vi "Initialize.vi"(0 "Gate Filter":bool, 1 "Gate Speed":dbl format="%.2f", 2 "Gate Dely":dbl format="%.2f", 3 "Gate Compliance (A)":dbl=0.001 format="%.2e", 4 "Drain Filter":bool, 5 "Drain Speed":dbl format="%.2f", 6 "Drain Delay":dbl format="%.2f", 7 "Drain Compliance (A)":dbl=0.001 format="%.2e") -> ()   [LabVIEW 2020]
panel:
  # "Initialize VI"
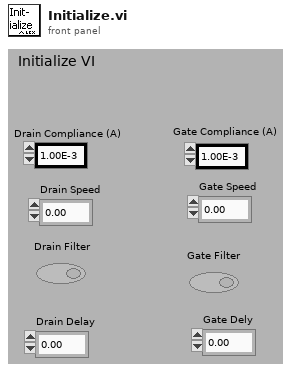
[diagram p1: front panel]
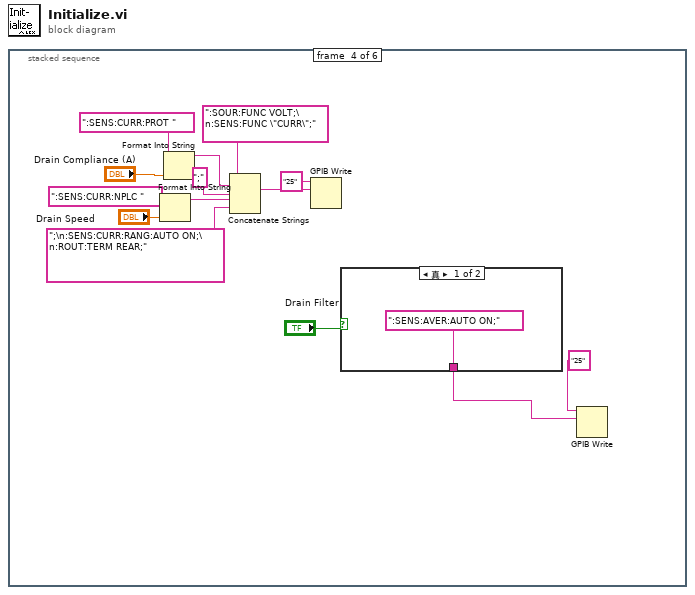
[diagram p0: block diagram]
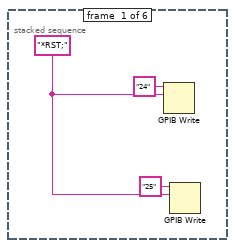
[diagram p2: hidden frame]
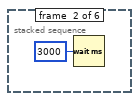
[diagram p3: hidden frame]
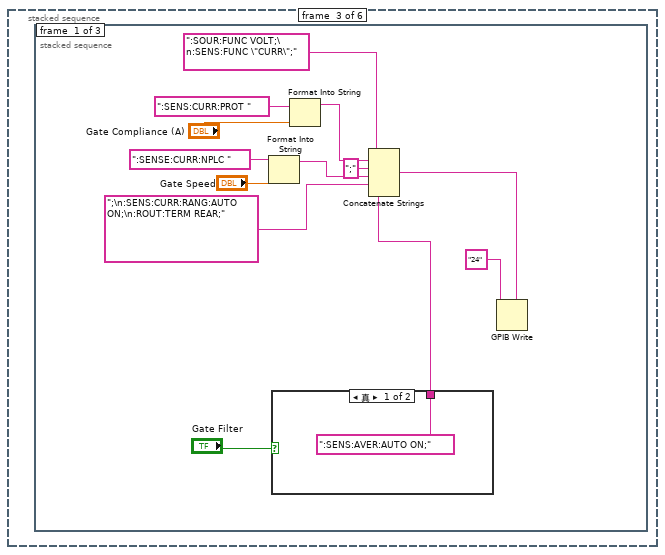
[diagram p4: hidden frame]
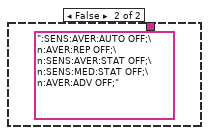
[diagram p5: hidden frame]
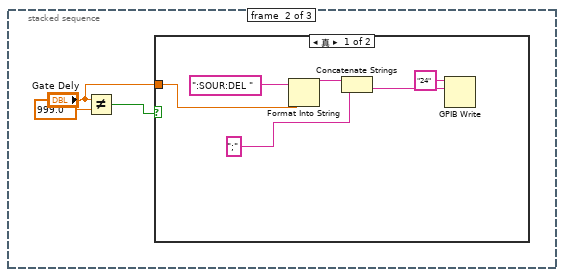
[diagram p6: hidden frame]
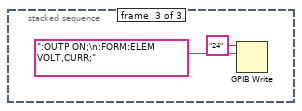
[diagram p8: hidden frame]
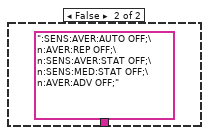
[diagram p9: hidden frame]
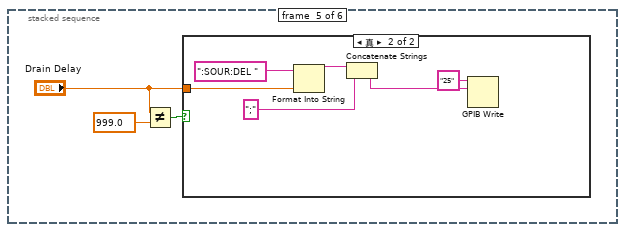
[diagram p10: hidden frame]
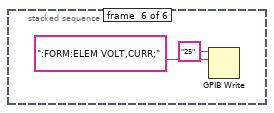
[diagram p12: hidden frame]
diagram:
  n1 = stacked-sequence {
    frame #0 {
      w1 = "*RST;"
      n2 = GPIB Write(0:"24" ("address string"), 1:w1) -> ()  [unwired: 3 in, 2 out]
      n3 = GPIB Write(0:"25" ("address string"), 1:w1) -> ()  [unwired: 3 in, 2 out]
    }
    frame #1 {
      n4 = Wait (ms)(milliseconds to wait=u32 3000) -> ()  [unwired: 1 out]
    }
    frame #2 {
      n5 = stacked-sequence {
        frame #0 {
          n6 = Format Into String(initial string=":SENSE:CURR:NPLC ", "Gate Speed") -> (resulting string=w6:string)  [unwired: 2 in, 1 out]
          n7 = case shown="真" "Gate Filter" {
            tunnel: [":SENS:AVER:AUTO ON;" ":SENS:AVER:AUTO OFF;\n:AVER:REP OFF;\n:SENS:AVER:STAT OFF;\n:SENS:MED:STAT OFF;\n:AVER:ADV OFF;"] -> w8
            frame True {
            }
            frame False {
            }
          }
          n8 = Format Into String(initial string=":SENS:CURR:PROT ", "Gate Compliance (A)") -> (resulting string=w13:string)  [unwired: 2 in, 1 out]
          n9 = Concatenate Strings(":SOUR:FUNC VOLT;\n:SENS:FUNC \"CURR\";", w13, ";" ("Substring"), w6, ";\n:SENS:CURR:RANG:AUTO ON;\n:ROUT:TERM REAR;", w8) -> (w15:string)
          n10 = GPIB Write(0:"24", 1:w15) -> ()  [unwired: 3 in, 2 out]
        }
        frame #1 {
          n11 = Not Equal?(x="Gate Dely", y=999.0) -> (x != y?=w21:bool)
          n12 = case shown="真" w21 {
            tunnel: "Gate Dely" -> [w25 _]
            frame True {
              n13 = Format Into String(initial string=":SOUR:DEL ", w25) -> (resulting string=w27:string)  [unwired: 2 in, 1 out]
              n14 = Concatenate Strings(w27, ";") -> (w24:string)
              n15 = GPIB Write(0:"24" ("address string"), 1:w24) -> ()  [unwired: 3 in, 2 out]
            }
            frame False {
            }
          }
        }
        frame #2 {
          n16 = GPIB Write(0:"24" ("address string"), 1:":OUTP ON;\n:FORM:ELEM VOLT,CURR;") -> ()  [unwired: 3 in, 2 out]
        }
      }
    }
    frame #3 {
      n17 = Format Into String(initial string=":SENS:CURR:NPLC ", "Drain Speed") -> (resulting string=w37:string)  [unwired: 2 in, 1 out]
      n18 = Format Into String(initial string=":SENS:CURR:PROT ", "Drain Compliance (A)") -> (resulting string=w41:string)  [unwired: 2 in, 1 out]
      n19 = Concatenate Strings(":SOUR:FUNC VOLT;\n:SENS:FUNC \"CURR\";", w41, ";", w37, ";\n:SENS:CURR:RANG:AUTO ON;\n:ROUT:TERM REAR;") -> (w32:string)
      n20 = GPIB Write(0:"25" ("address string"), 1:w32) -> ()  [unwired: 3 in, 2 out]
      n21 = case shown="真" "Drain Filter" {
        tunnel: [":SENS:AVER:AUTO ON;" ":SENS:AVER:AUTO OFF;\n:AVER:REP OFF;\n:SENS:AVER:STAT OFF;\n:SENS:MED:STAT OFF;\n:AVER:ADV OFF;"] -> w31
        frame True {
        }
        frame False {
        }
      }
      n22 = GPIB Write(0:"25", 1:w31) -> ()  [unwired: 3 in, 2 out]
    }
    frame #4 {
      n23 = Not Equal?(x="Drain Delay", y=999.0) -> (x != y?=w49:bool)
      n24 = case shown="真" w49 {
        tunnel: "Drain Delay" -> [_ w54]
        frame False {
        }
        frame True {
          n25 = Format Into String(initial string=":SOUR:DEL ", w54) -> (resulting string=w55:string)  [unwired: 2 in, 1 out]
          n26 = Concatenate Strings(w55, ";") -> (w51:string)
          n27 = GPIB Write(0:"25" ("address string"), 1:w51) -> ()  [unwired: 3 in, 2 out]
        }
      }
    }
    frame #5 {
      n28 = GPIB Write(0:"25" ("address string"), 1:":FORM:ELEM VOLT,CURR;") -> ()  [unwired: 3 in, 2 out]
    }
  }
